vi "fromXml.vi"(8 "error in (no error)":errorcluster, 10 "dataPointXml":refnum<class "xmlNode.lvclass">, 11 "Delay in":refnum<class "Delay.lvclass">) -> (0 "error out":errorcluster, 3 "Delay out":refnum<class "Delay.lvclass">)   [LabVIEW 2009]
uses:
  ScriptEvent.lvclass
  xmlNode/xmlNode.lvclass
  Delay.lvclass
panel:
  # "not used\n\nreadInNativeXML instead"
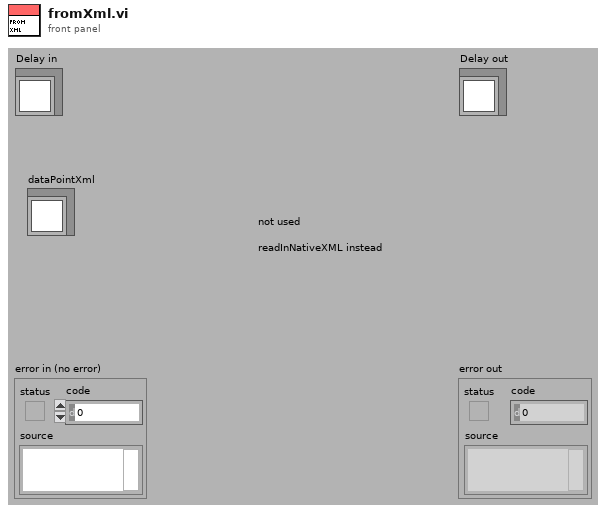
[diagram p1: front panel]
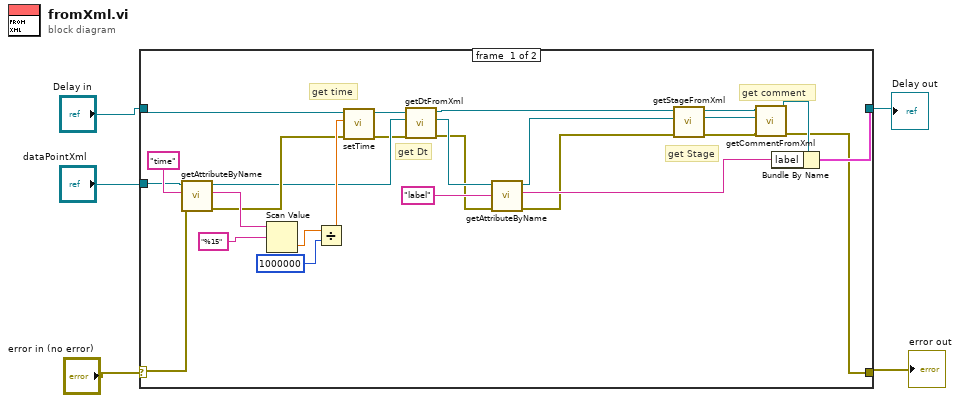
[diagram p0: block diagram]
diagram:
  n1 = case shown="No Error" "error in (no error)" {
    selector: "error in (no error)" -> [w21 w33]
    tunnel: [w7 w33] -> w2
    tunnel: [w10 w32] -> w1
    tunnel: "Delay in" -> [w20 w32]
    tunnel: "dataPointXml" -> [w22 _]
    frame #0 {
      # "get comment"
      # "get Stage"
      # "get Dt"
      # "get time"
      n2 = call-dynamic "getAttributeByName.vi"("error in (no error)"=w21, "AttributeName"="time", "xmlNode in"=w22) -> ("error out"=w18:errorcluster, "attribute string"=w27:string, "xmlNode out"=w17:refnum<class "xmlNode.lvclass">)  [unwired: 6 in]
      n3 = Scan Value(string=w27, format string="%15") -> (value=w25:dbl)  [unwired: 1 in, 1 out]
      n4 = Divide(x=w25, y=1000000) -> (x/y=w23:dbl)
      n5 = call "setTime.vi"("error in (no error)"=w18, "time"=w23, "ScriptEvent.lvclass in"=w20) -> ("error out"=w16:errorcluster, "ScriptEvent.lvclass out"=w19:refnum<class "Delay.lvclass">)  [unwired: 7 in]
      n6 = call "getDtFromXml.vi"("error in (no error)"=w16, "Xml"=w17, "ScriptEvent in"=w19) -> ("error out"=w12:errorcluster, "Xml out"=w15:refnum<class "xmlNode.lvclass">, "ScriptEvent out"=w6:refnum<class "Delay.lvclass">)  [unwired: 6 in]
      n7 = call-dynamic "getAttributeByName.vi"("error in (no error)"=w12, "AttributeName"="label", "xmlNode in"=w15) -> ("error out"=w8:errorcluster, "attribute string"=w9:string, "xmlNode out"=w13:refnum<class "xmlNode.lvclass">)  [unwired: 6 in]
      n8 = call "getStageFromXml.vi"("error in (no error)"=w8, "Xml"=w13, "ScriptEvent in"=w6) -> ("error out"=w29:errorcluster, "Xml out"=w30:refnum<class "xmlNode.lvclass">, "ScriptEvent out"=w31:refnum<class "Delay.lvclass">)  [unwired: 6 in]
      n9 = call "getCommentFromXml.vi"("error in (no error)"=w29, "Xml"=w30, "ScriptEvent in"=w31) -> ("error out"=w7:errorcluster, "ScriptEvent out"=w11:refnum<class "Delay.lvclass">)  [unwired: 6 in, 1 out]
      n10 = Bundle By Name(cluster=w11, "label"=w9) -> (w10:cluster{})
    }
    frame #1 {
    }
  }
  "error out" <- w2
  "Delay out" <- w1
